vi "New_Magazine_Test.vi"(11 "Joystick_In":T1={"Pilot Left Joystick X"=0.07086614173228346, "Pilot Left Joystick Y"=-0.047244094488188976, "Pilot A Button"=FALSE, "Pilot B Button"=FALSE, "Pilot X Button"=FALSE, "Pilot Y Button"=FALSE, "Pilot Left Bumper"=FALSE, "Pilot Right Bumper"=FALSE, "Pilot View Button"=FALSE, "Pilot Menu Button"=FALSE, "Pilot Left Joystick Press"=FALSE, "Pilot Right Joystick Press"=FALSE, "Pilot Left Trigger"=0.0, "Pilot Right Joystick X"=-0.047244094488188976, "Pilot Right Joystick Y"=0.03937007874015748, "Pilot Right Trigger"=0.0, "Copilot Left Joystick X"=0.047244094488188976, "Copilot Left Joystick Y"=0.023622047244094488, "Copilot A Button"=FALSE, "Copilot B Button"=FALSE, "Copilot X Button"=FALSE, "Copilot Y Button"=FALSE, "Copilot Left Bumper"=FALSE, "Copilot Right Bumper"=FALSE, "Copilot View Button"=FALSE, "Copilot Menu Button"=FALSE, "Copilot Left Joystick Press"=FALSE, "Copilot Right Joystick Press"=FALSE, "Copilot Left Trigger"=0.0, "Copilot Right Joystick X"=-0.015748031496062992, "Copilot Right Joystick Y"=0.047244094488188976, "Copilot Right Trigger"=0.0, "Pilot D-pad North"=FALSE, "Pilot D-pad South"=FALSE, "Pilot D-pad East"=FALSE, "Pilot D-pad West"=FALSE, "Pilot D-pad NE "=FALSE, "Pilot D-pad SE"=FALSE, "Pilot D-pad SW"=FALSE, "Pilot D-pad NW"=FALSE, "CoPilot D-pad North"=FALSE, "CoPilot D-pad South"=FALSE, "CoPilot D-pad East"=FALSE, "CoPilot D-pad West"=FALSE, "CoPilot D-pad NE"=FALSE, "CoPilot D-pad SE"=FALSE, "CoPilot D-pad SW"=FALSE, "CoPilot D-pad NW"=FALSE, "Pilot Left Trigger Pressed"=FALSE, "Pilot Right Trigger Pressed"=FALSE, "CoPilot Left Trigger Pressed"=FALSE, "CoPilot Right Trigger Pressed"=FALSE}) -> ()   [LabVIEW 2019]
uses:
  Utility_VIs/Joystick_Controls.ctl
  New_Magazine_Cluster.ctl
  New_Magazine_Control_States.ctl
  New_Magazine_Globals.vi
panel:
  in  "Magazine Power":dbl=0.9
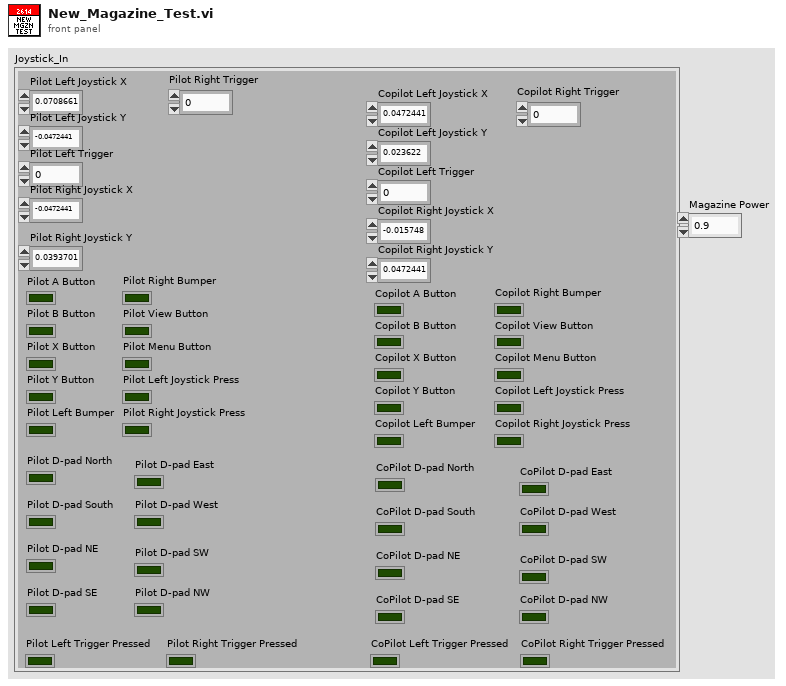
[diagram p1: front panel]
types:
  T1 = typedef "Joystick_Controls.ctl" = cluster{"Pilot Left Joystick X":dbl, "Pilot Left Joystick Y":dbl, "Pilot A Button":bool, "Pilot B Button":bool, "Pilot X Button":bool, "Pilot Y Button":bool, "Pilot Left Bumper":bool, "Pilot Right Bumper":bool, "Pilot View Button":bool, "Pilot Menu Button":bool, "Pilot Left Joystick Press":bool, "Pilot Right Joystick Press":bool, "Pilot Left Trigger":dbl, "Pilot Right Joystick X":dbl, "Pilot Right Joystick Y":dbl, "Pilot Right Trigger":dbl, "Copilot Left Joystick X":dbl, "Copilot Left Joystick Y":dbl, "Copilot A Button":bool, "Copilot B Button":bool, "Copilot X Button":bool, "Copilot Y Button":bool, "Copilot Left Bumper":bool, "Copilot Right Bumper":bool, "Copilot View Button":bool, "Copilot Menu Button":bool, "Copilot Left Joystick Press":bool, "Copilot Right Joystick Press":bool, "Copilot Left Trigger":dbl, "Copilot Right Joystick X":dbl, "Copilot Right Joystick Y":dbl, "Copilot Right Trigger":dbl, "Pilot D-pad North":bool, "Pilot D-pad South":bool, "Pilot D-pad East":bool, "Pilot D-pad West":bool, "Pilot D-pad NE ":bool, "Pilot D-pad SE":bool, "Pilot D-pad SW":bool, "Pilot D-pad NW":bool, "CoPilot D-pad North":bool, "CoPilot D-pad South":bool, "CoPilot D-pad East":bool, "CoPilot D-pad West":bool, "CoPilot D-pad NE":bool, "CoPilot D-pad SE":bool, "CoPilot D-pad SW":bool, "CoPilot D-pad NW":bool, "Pilot Left Trigger Pressed":bool, "Pilot Right Trigger Pressed":bool, "CoPilot Left Trigger Pressed":bool, "CoPilot Right Trigger Pressed":bool}
  T2 = typedef "New_Magazine_Cluster.ctl" = cluster{"Control_States":T3, "Firing":bool, "Throttle":dbl, "Spinning Up":bool, "Off":bool, "Extend_Magazine_Manual":bool}
  T3 = typedef "New_Magazine_Control_States.ctl" = enum16{"No-Op", "Up", "Down", "Manual", "Fire", "Spinning Up"}
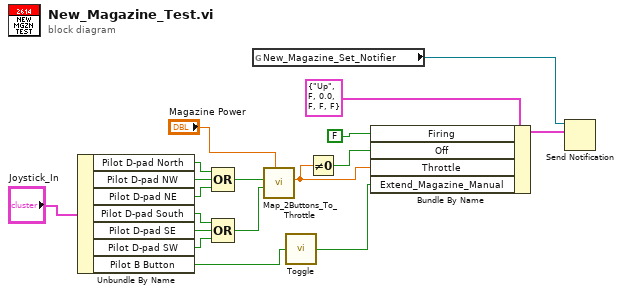
[diagram p0: block diagram]
diagram:
  n1 = Unbundle By Name("Joystick_In") -> ("Pilot D-pad North"=w10:bool, "Pilot D-pad NW"=w9:bool, "Pilot D-pad NE"=w8:bool, "Pilot D-pad South"=w6:bool, "Pilot D-pad SE"=w5:bool, "Pilot D-pad SW"=w4:bool, "Pilot B Button"=w1:bool)
  n2 = Compound Arithmetic op=OR(w10, w9, w8) -> (w7:bool)
  n3 = Compound Arithmetic op=OR(w6, w5, w4) -> (w3:bool)
  n4 = global read "New_Magazine_Globals.vi" "New_Magazine_Set_Notifier"() -> (w14:refnum<notifier>)
  n5 = call "Map_2Buttons_To_Throttle.vi"("Power"="Magazine Power", "Down"=w3, "Up"=w7) -> ("Throttle"=w11:dbl)  [unwired: 8 in]
  n6 = call "Toggle.vi"("Boolean"=w1) -> ("Boolean Out"=w2:bool)
  n7 = Not Equal To 0?(x=w11) -> (x != 0?=w12:bool)
  n8 = Bundle By Name(cluster=T2 {"Control_States"=enum."Up", "Firing"=FALSE, "Throttle"=0.0, "Spinning Up"=FALSE, "Off"=FALSE, "Extend_Magazine_Manual"=FALSE} ("New_Magazine"), "Firing"=FALSE, "Off"=w12, "Throttle"=w11, "Extend_Magazine_Manual"=w2) -> (w15:T2)
  n9 = Send Notification(notification=w15, notifier=w14) -> ()  [unwired: 1 in, 2 out]
